vi "Crop Map.vi"(8 "error in (no error)":errorcluster, 11 "Map Model in":refnum<class "Map Model.lvclass">) -> (0 "error out":errorcluster, 3 "Map Model out":refnum<class "Map Model.lvclass">)   [LabVIEW 2020, in "Map Model.lvlib" / "Map Model.lvclass"]
uses:
  Map Model.lvclass
  Map Model.lvclass/Map Model.ctl
  Stack/Stack.lvclass
panel:
  # "NOTICE -- YOU MUST LEAVE THIS NOTICE IN PLACE.\n\nCopyright (c) 2017, LIANG LIU Shawn.Liu.cn@gmail.com\nAll rights reserved.\n\nRedistribution and use in source and binary forms, with or without modification, are permitted provided that the following conditions are met:\n-Redistributions of source code must retain the above copyright notice, this list of conditions and the following disclaimer.\n-Redistributions in binary form must reproduce the above copyright notice, this list of conditions and the following disclaimer in the documentation and/or other materials provided with the distribution.\n-Neither the name of the eLp nor the names of its contributors may be used to endorse or promote products derived from this software without specific prior written permission.\n\nTHIS SOFTWARE IS PROVIDED BY THE COPYRIGHT HOLDERS AND CONTRIBUTORS \"AS IS\" AND ANY EXPRESS OR IMPLIED WARRANTIES, INCLUDING, BUT NOT LIMITED TO, THE IMPLIED WARRANTIES OF MERCHANTABILITY AND FITNESS FOR A PARTICULAR PURPOSE ARE DISCLAIMED. IN NO EVENT SHALL THE COPYRIGHT HOLDER OR CONTRIBUTORS BE LIABLE FOR ANY DIRECT, INDIRECT, INCIDENTAL, SPECIAL, EXEMPLARY, OR CONSEQUENTIAL DAMAGES (INCLUDING, BUT NOT LIMITED TO, PROCUREMENT OF SUBSTITUTE GOODS OR SERVICES; LOSS OF USE, DATA, OR PROFITS; OR BUSINESS INTERRUPTION) HOWEVER CAUSED AND ON ANY THEORY OF LIABILITY, WHETHER IN CONTRACT, STRICT LIABILITY, OR TORT (INCLUDING NEGLIGENCE OR OTHERWISE) ARISING IN ANY WAY OUT OF THE USE OF THIS SOFTWARE, EVEN IF ADVISED OF THE POSSIBILITY OF SUCH DAMAGE."
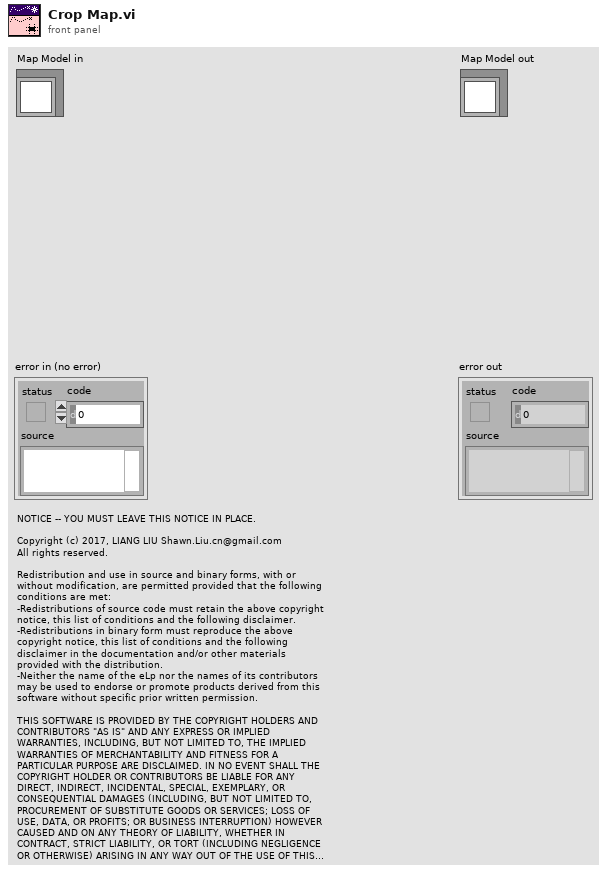
[diagram p1: front panel]
types:
  T1 = enum8{"Enabled", "Disabled", "Disabled and Grayed Out"}
  T2 = typedef "LVPointTypeDef.ctl" = cluster{"Horizontal":i16, "Vertical":i16}
  T3 = typedef "imagedata.ctl" = cluster{"image type":i32, "image depth":i32, "image":u8[], "mask":u8[], "colors":u32[], "Rectangle":cluster{"left":i16, "top":i16, "right":i16, "bottom":i16}}
  T4 = cluster{"left":i16, "top":i16, "right":i16, "bottom":i16}
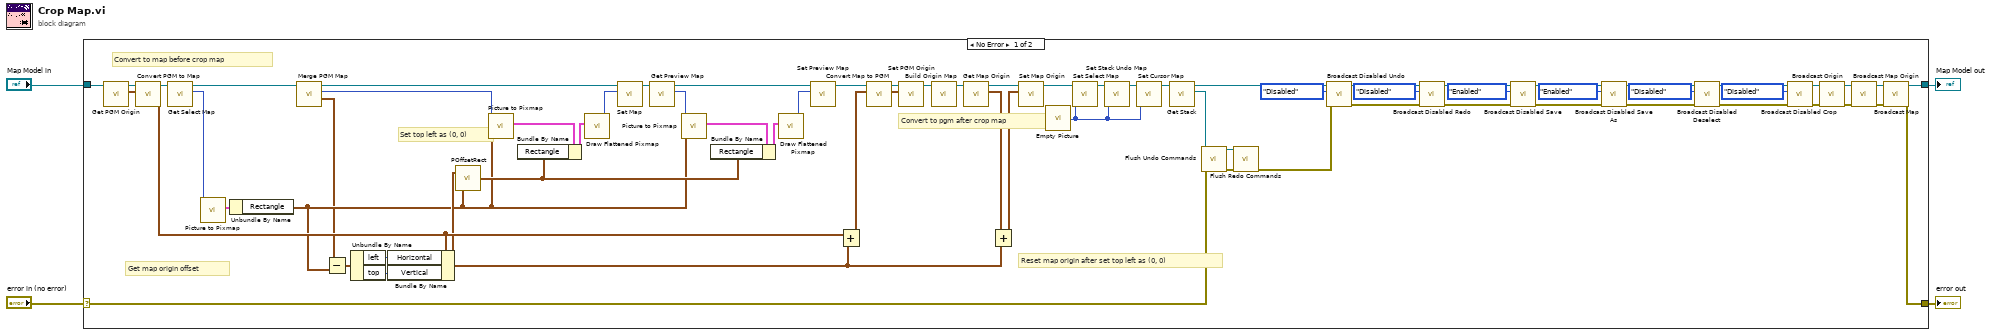
[diagram p0: block diagram]
diagram:
  n1 = case shown="No Error" "error in (no error)" {
    selector: "error in (no error)" -> [w72 w76]
    tunnel: [w74 w75] -> w4
    tunnel: [w73 w76] -> w3
    tunnel: "Map Model in" -> [w29 w75]
    frame No Error {
      # "Reset map origin after set top left as (0, 0)"
      # "Convert to pgm after crop map"
      # "Convert to map before crop map"
      # "Set top left as (0, 0)"
      # "Get map origin offset"
      n2 = call "Get PGM Origin.vi"("Map Model in"=w29) -> ("PGM Origin"=w42:cluster{"Horizontal":dbl, "Vertical":dbl}, "Map Model out"=w43:refnum<class "Map Model.lvclass">)  [unwired: 9 in]
      n3 = call "Convert PGM to Map.vi"("Position on PGM"=w42, "Map Model in"=w43) -> ("Position on Map"=w35:T2, "Map Model out"=w31:refnum<class "Map Model.lvclass">)  [unwired: 8 in]
      n4 = call "Get Select Map.vi"("Map Model in"=w31) -> ("Select Map"=w17:picture, "Map Model out"=w69:refnum<class "Map Model.lvclass">)  [unwired: 9 in]
      n5 = call <vilib>:"Picture to Pixmap.vi"("picture"=w17) -> ("image data"=w71:T3)  [unwired: 9 in, 1 out]
      n6 = Unbundle By Name(w71) -> ("Rectangle"=w16:T4)
      n7 = call "Merge PGM Map.vi"("Map Model in"=w69) -> ("Map Rectangle"=w15:T4, "Map"=w70:picture, "Map Model out"=w67:refnum<class "Map Model.lvclass">)  [unwired: 7 in, 1 out]
      n8 = Subtract(x=w15, y=w16) -> (x-y=w19:T4)
      n9 = Unbundle By Name(w19) -> ("left"=w34:i16, "top"=w33:i16)
      n10 = Bundle By Name(cluster=w35, "Horizontal"=w34, "Vertical"=w33) -> (w18:T2)
      n11 = call <vilib>:"POffsetRect.vi"("rect"=w16, "point"=w18) -> ("offset rect"=w26:T4)
      n12 = call <vilib>:"Picture to Pixmap.vi"("rect"=w16, "picture"=w70) -> ("image data"=w68:T3)  [unwired: 8 in, 1 out]
      n13 = Bundle By Name(cluster=w68, "Rectangle"=w26) -> (w28:T3)
      n14 = call <vilib>:"Draw Flattened Pixmap.vi"("image data"=w28) -> ("new picture"=w66:picture)  [unwired: 8 in]
      n15 = call "Set Map.vi"("Map"=w66, "Map Model in"=w67) -> ("Map Model out"=w64:refnum<class "Map Model.lvclass">)  [unwired: 9 in]
      n16 = call "Get Preview Map.vi"("Map Model in"=w64) -> ("Preview Map"=w14:picture, "Map Model out"=w65:refnum<class "Map Model.lvclass">)  [unwired: 9 in]
      n17 = call <vilib>:"Picture to Pixmap.vi"("rect"=w16, "picture"=w14) -> ("image data"=w63:T3)  [unwired: 8 in, 1 out]
      n18 = Bundle By Name(cluster=w63, "Rectangle"=w26) -> (w27:T3)
      n19 = call <vilib>:"Draw Flattened Pixmap.vi"("image data"=w27) -> ("new picture"=w62:picture)  [unwired: 8 in]
      n20 = call "Set Preview Map.vi"("Preview Map"=w62, "Map Model in"=w65) -> ("Map Model out"=w30:refnum<class "Map Model.lvclass">)  [unwired: 9 in]
      n21 = Add(x=w35, y=w18) -> (x+y=w32:T2)
      n22 = call "Convert Map to PGM.vi"("Position on Map"=w32, "Map Model in"=w30) -> ("Position on PGM"=w40:T2, "Map Model out"=w53:refnum<class "Map Model.lvclass">)  [unwired: 8 in]
      n23 = call "Set PGM Origin.vi"("PGM Origin"=w40, "Map Model in"=w53) -> ("Map Model out"=w41:refnum<class "Map Model.lvclass">)  [unwired: 9 in]
      n24 = call "Build Origin Map.vi"("Map Model in"=w41) -> ("Map Model out"=w39:refnum<class "Map Model.lvclass">)  [unwired: 9 in, 1 out]
      n25 = call "Get Map Origin.vi"("Map Model in"=w39) -> ("Map Origin"=w20:T2, "Map Model out"=w25:refnum<class "Map Model.lvclass">)  [unwired: 9 in]
      n26 = Add(x=w20, y=w18) -> (x+y=w13:T2)
      n27 = call "Set Map Origin.vi"("Map Origin"=w13, "Map Model in"=w25) -> ("Map Model out"=w24:refnum<class "Map Model.lvclass">)  [unwired: 9 in]
      n28 = call "Empty Picture"() -> ("empty picture"=w45:picture)
      n29 = call "Set Select Map.vi"("Select Map"=w45, "Map Model in"=w24) -> ("Map Model out"=w38:refnum<class "Map Model.lvclass">)  [unwired: 9 in]
      n30 = call "Set Stack Undo Map.vi"("Stack Undo Map"=w45, "Map Model in"=w38) -> ("Map Model out"=w61:refnum<class "Map Model.lvclass">)  [unwired: 9 in]
      n31 = call "Set Cursor Map.vi"("Cursor Map"=w45, "Map Model in"=w61) -> ("Map Model out"=w44:refnum<class "Map Model.lvclass">)  [unwired: 9 in]
      n32 = call "Get Stack.vi"("Map Model in"=w44) -> ("Stack"=w54:refnum<class "Stack.lvclass">, "Map Model out"=w56:refnum<class "Map Model.lvclass">)  [unwired: 9 in]
      n33 = call "Flush Undo Commands.vi"("error in (no error)"=w72, "Stack in"=w54) -> ("error out"=w37:errorcluster, "Stack out"=w60:refnum<class "Stack.lvclass">)  [unwired: 8 in]
      n34 = call "Flush Redo Commands.vi"("error in (no error)"=w37, "Stack in"=w60) -> ("error out"=w36:errorcluster)  [unwired: 8 in, 1 out]
      n35 = call "Broadcast Disabled Undo.vi"("error in (no error)"=w36, "Disabled Undo"=T1."Disabled", "Map Model in"=w56) -> ("error out"=w55:errorcluster, "Map Model out"=w59:refnum<class "Map Model.lvclass">)  [unwired: 7 in]
      n36 = call "Broadcast Disabled Redo.vi"("error in (no error)"=w55, "Disabled Redo"=T1."Disabled", "Map Model in"=w59) -> ("error out"=w51:errorcluster, "Map Model out"=w48:refnum<class "Map Model.lvclass">)  [unwired: 7 in]
      n37 = call "Broadcast Disabled Save.vi"("error in (no error)"=w51, "Disabled Save"=T1."Enabled", "Map Model in"=w48) -> ("error out"=w50:errorcluster, "Map Model out"=w52:refnum<class "Map Model.lvclass">)  [unwired: 7 in]
      n38 = call "Broadcast Disabled Save As.vi"("error in (no error)"=w50, "Disabled Save As"=T1."Enabled", "Map Model in"=w52) -> ("error out"=w7:errorcluster, "Map Model out"=w8:refnum<class "Map Model.lvclass">)  [unwired: 7 in]
      n39 = call "Broadcast Disabled Deselect.vi"("error in (no error)"=w7, "Disabled Deselect"=T1."Disabled", "Map Model in"=w8) -> ("error out"=w9:errorcluster, "Map Model out"=w12:refnum<class "Map Model.lvclass">)  [unwired: 7 in]
      n40 = call "Broadcast Disabled Crop.vi"("error in (no error)"=w9, "Disabled Crop"=T1."Disabled", "Map Model in"=w12) -> ("error out"=w5:errorcluster, "Map Model out"=w6:refnum<class "Map Model.lvclass">)  [unwired: 7 in]
      n41 = call "Broadcast Origin.vi"("error in (no error)"=w5, "Map Model in"=w6) -> ("error out"=w49:errorcluster, "Map Model out"=w22:refnum<class "Map Model.lvclass">)  [unwired: 8 in]
      n42 = call "Broadcast Map Origin.vi"("error in (no error)"=w49, "Map Model in"=w22) -> ("error out"=w23:errorcluster, "Map Model out"=w21:refnum<class "Map Model.lvclass">)  [unwired: 8 in]
      n43 = call "Broadcast Map.vi"("error in (no error)"=w23, "Map Model in"=w21) -> ("error out"=w73:errorcluster, "Map Model out"=w74:refnum<class "Map Model.lvclass">)  [unwired: 8 in]
    }
    frame Error {
    }
  }
  "error out" <- w3
  "Map Model out" <- w4
